vi "Valid Measurement Client Name.vi"(8 "error in":errorcluster, 10 "requested client name":string, 11 "library names":string[](array[string])) -> (0 "error out":errorcluster, 3 "valid name?":bool)   [LabVIEW 2021, in "NI Measurement V2 Client Generator Runtime.lvlib"]
uses:
  NI Measurement V2 Client Generator Runtime.lvlib
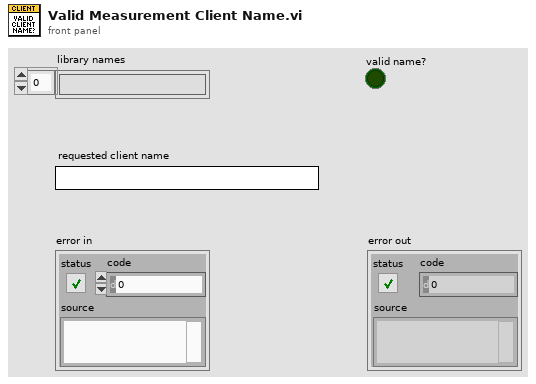
[diagram p1: front panel]
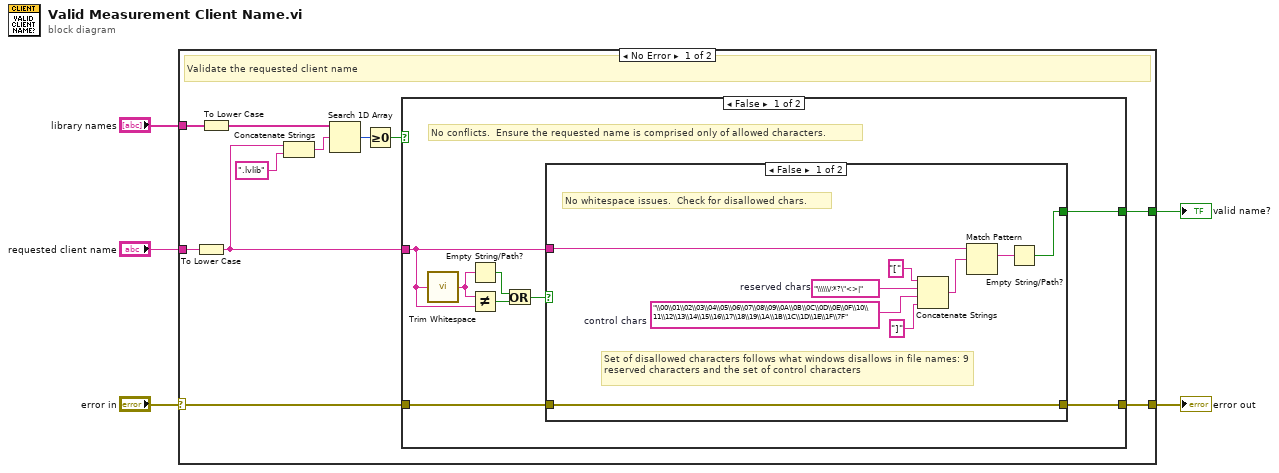
[diagram p0: block diagram]
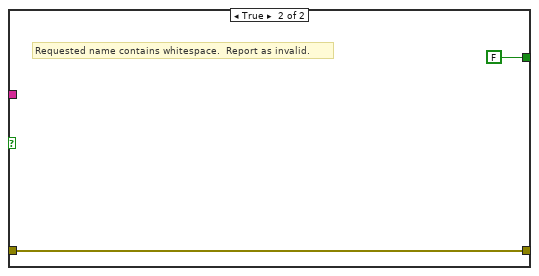
[diagram p2: hidden frame]
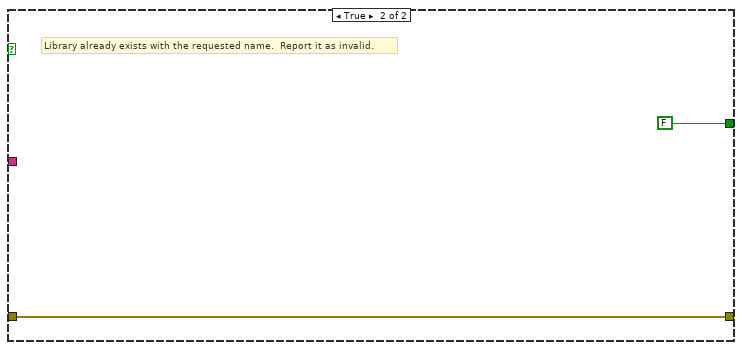
[diagram p3: hidden frame]
diagram:
  n1 = case shown="No Error" "error in" {
    selector: "error in" -> [w13 w38]
    tunnel: "requested client name" -> [w16 _]
    tunnel: [w15 w38] -> w4
    tunnel: [w14 _] -> w3
    tunnel: "library names" -> [w10 _]
    frame No Error {
      # "Validate the requested client name"
      n2 = To Lower Case(string=w16) -> (all lower case string=w7:string)
      n3 = To Lower Case(string=w10) -> (all lower case string=w9:string[])
      n4 = Concatenate Strings(w7, ".lvlib" ("string")) -> (w8:string)
      n5 = Search 1D Array(1D array=w9, element=w8) -> (index of element=w12:i32)  [unwired: 1 in]
      n6 = Greater Or Equal To 0?(x=w12) -> (x >= 0?=w11:bool)
      n7 = case shown="False" w11 {
        tunnel: w13 -> [w24 w37]
        tunnel: [w23 w37] -> w15
        tunnel: [w22 FALSE ("Valid Name?")] -> w14
        tunnel: w7 -> [w18 _]
        frame False {
          # "No conflicts.  Ensure the requested name is comprised only of allowed characters."
          n8 = call <vilib>:"Trim Whitespace.vi"("string"=w18) -> ("trimmed string"=w21:string)  [unwired: 1 in]
          n9 = Empty String/Path?(string/path=w21) -> (empty?=w19:bool)
          n10 = Not Equal?(x=w21, y=w18) -> (x != y?=w20:bool)
          n11 = Or(x=w19, y=w20) -> (x .or. y?=w17:bool)
          n12 = case shown="False" w17 {
            tunnel: w18 -> [w32 _]
            tunnel: w24 -> [w33 w35]
            tunnel: [w33 w35] -> w23
            tunnel: [w30 FALSE] -> w22
            frame False {
              w25 = "\\00\\01\\02\\03\\04\\05\\06\\07\\08\\09\\0A\\0B\\0C\\0D\\0E\\0F\\10\\11\\12\\13\\14\\15\\16\\17\\18\\19\\1A\\1B\\1C\\1D\\1E\\1F\\7F"  # control chars
              w29 = "\\\\\\/:*?\"<>|"  # reserved chars
              # "Set of disallowed characters follows what windows disallows in file names: 9 reserved characters and the set of control characters"
              # "No whitespace issues.  Check for disallowed chars."
              n13 = Concatenate Strings("[" ("string"), w29, w25, "]" ("string")) -> (w26:string)
              n14 = Match Pattern(string=w32, regular expression=w26) -> (match substring=w31:string)  [unwired: 1 in, 3 out]
              n15 = Empty String/Path?(string/path=w31) -> (empty?=w30:bool)
            }
            frame True {
              # "Requested name contains whitespace.  Report as invalid."
            }
          }
        }
        frame True {
          # "Library already exists with the requested name.  Report it as invalid."
        }
      }
    }
    frame Error {
      # "Pass"
    }
  }
  "error out" <- w4
  "valid name?" <- w3
